vi "optionsAcq_gainOpticalDetector.vi"(0 "reference":refnum<class "OSA300.lvclass">, 2 "gain_idx":u16=1, 4 "readWrite":enum16{"read", "write"}(ring), 5 "error in (no error)":errorcluster, 7 "ignore range violation (false)":bool) -> (14 "duplicate reference":refnum<class "OSA300.lvclass">, 15 "status":string, 16 "gain_idx  out":u16, 17 "gain_relative":dbl, 19 "error out":errorcluster)   [LabVIEW 2010, in "OSA300.lvclass"]
uses:
  OSA300.lvclass
  _OSAchannel_class/OSAchannel.lvclass
  OSA.lvclass
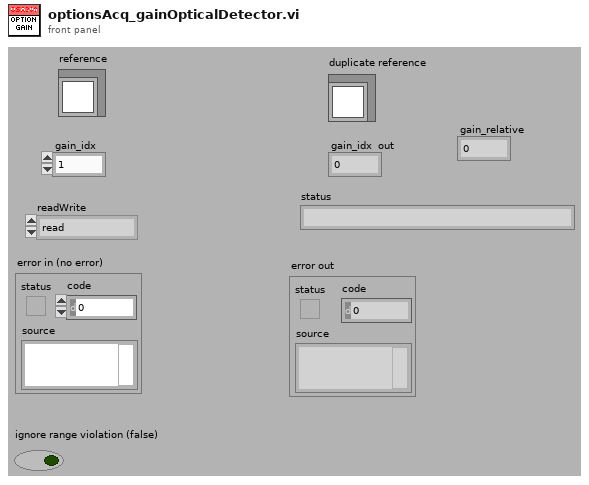
[diagram p1: front panel]
types:
  T1 = typedef "OSA20X_misc.lvlib/amplifier_sort.ctl" = enum16{"amp_unknown", "amp_se_8", "amp_se_12_lg", "amp_se_12", "amp_se_16", "amp_diff_8", "amp_diff_12_lg", "amp_diff_12_ir", "amp_diff_16", "amp_other", "amp_other_2"}
  T2 = typedef "OSA20X_misc.lvlib/detector_sort.ctl" = enum16{"unknown", "Silicon", "Silicon PIN", "Silicon MPPC", "InGaAs", "InGaAs ext low", "InGaAs ext high", "InAs", "InAsSb", "InSb", "MCT", "other", "other2", "other3"}
  T3 = typedef "OSA20X_misc.lvlib/interferogram_smoothing.ctl" = enum16{"NONE", "BINOMIAL", "SAVITSKY_GOLAY", "FOURIER", "MOVING_AVERAGE", "GAUSSIAN"}
  T4 = typedef "OSA20X_misc.lvlib/PDTemperatureMode.ctl" = enum16{"cool: better sensitivity/noise floor", "warm: extended wl range"}
  T5 = cluster{"waveMin (cm-1)":sgl, "waveMax (cm-1)":sgl, "gainOffset_auto":bool, "gain":i32, "gain levels nr":u16, "offset":i32, "offset max":u16, "damper available":bool, "damper active":bool, "amplifier sort":T1, "detector sort":T2, "channelIdx global":u16, "spectrIdx":u16, "waveMeter on":bool, "ref gainLevels rel.":refnum<data-value>, "intfgrm_smooth_width":u16, "intfgrm_smooth_nrOfPasses":u16, "intfgrm_smooth":T3, "adc #bits":u16, "temp Variable":bool, "spectr_smooth":T3, "spectr_smooth_width":u16, "spectr_smooth_nrOfPasses":u16, "PD sensitivity mode":T4, "damper auto":bool}
  T6 = typedef "OSA.lvclass/ObjectAttributes.ctl" = cluster{"Stop":bool, "dataType":T7, "spectrometerIdx":u16, "buffer size interferogram":i32, "interferogram":cluster{"new":bool, "plot_x_ min":sgl, "plot_x_max":sgl, "plot_y_min":sgl, "plot_y_max":sgl, "Graph Intrfrgrm":T8, "timeStamp":u32, "signal (%)":dbl, "traces":cluster{"idx":u32, "broadBand":bool, "monoChromatic":bool, "peakToPeakSignal":dbl, "peakToPeakPos":dbl}[], "traces idx last":i32}, "spectrum":cluster{"new":bool, "plot_x_min":sgl, "plot_x_max":sgl, "plot_unit_x":T9, "plot_unit_y":T10, "plot_y_min":sgl, "plot_y_max":sgl, "Graph Spectrum":T8, "timeStamp":u32, "X_VAL_OPTIONS":enum16{"MIN_MAX", "ARRAY"}, "traces":cluster{"idx":u32}[], "traces idx last":i32}, "Thorlabs_OSA_64.lvclass:queue_action.ctlqueue ref":refnum<queue>, "action":T11, "plot zoom step":dbl, "buffer semaphore":T12, "acq stopped":bool, "dataType active":T7, "temperature (degr C)":sgl, "pressure (hPa)":sgl, "rel humidity (%)":sgl, "settings":cluster{"resolution":u16, "sensitivity":u16, "Average":bool, "average nr":u32, "apodisation":T13, "acq delay (ms)":u32, "airMesure":T14, "wmtr on":bool, "intfgrm_smooth_width":u16, "intfgrm_smooth_nrOfPasses":u16, "intfgrm_smooth":T3, "phaseCorrection":T15, "zeroFill":u8, "spectr_smooth":T3, "spectr_smooth_width":u16, "spectr_smooth_nrOfPasses":u16, "resolution (/cm)":sgl, "REF wavelength, (nm)":dbl, "gain_idx":u16, "gainAuto":bool, "gain_relative":dbl, "PD sensitivity mode":T4, "PD senseMode implemented":bool, "SensorTemperature implemented":bool, "SensorPressure implemented":bool, "SensorHumidity implemented":bool, "attenuationAuto":bool, "attenuationOnOff":bool, "attenuationAvailable":bool, "offsetAvailable":bool, "offset":i32, "offset max":u16}, "peaks position":sgl[], "peaks width":sgl[], "peaks height":sgl[], "peaks max nr":u32, "peaks latest nr":i32, "peaks new":bool, "power":dbl, "power new":bool, "path":string, "wavelength (WNr)":dbl, "wavelength new":bool, "buffer size spectrum":i32, "status":string, "vi reference":refnum<vi>, "funcPointer":u64, "libraryPointer":u64, "singleAcquisition":bool, "coherenceLength (cm)":dbl, "coherenceLength new":bool, "spectrometer model":string, "spectrometer serial nr":string, "peaks thld left":sgl[], "peaks thld right":sgl[], "coherenceLength error (cm)":dbl, "ADC bits":u16, "peaks position centroid":sgl[], "peaks height centroid":sgl[], "OSA series":T16, "channel index spectrum":u16, "spectrometer rangeLow, (/cm)":dbl, "spectrometer rangeHigh, (/cm)":dbl, "channel index interferogram":u16}
  T7 = typedef "OSA.lvclass/acq_dataType.ctl" = enum16{"none", "interferogram", "spectrum"}
  T8 = typedef "OSA.lvclass/graph_intensity.ctl" = refnum<vi>
  T9 = typedef "OSA.lvclass/spectrum_x_unit.ctl" = enum16{"wavenr/cm", "THz", "eV", "nm_air", "nm_vac"}
  T10 = typedef "OSA.lvclass/y_unit.ctl" = enum16{"ADC counts", "dBm pwr absolute", "dBm pwr density", "mW pwr absolute", "mW pwr density"}
  T11 = typedef "OSA.lvclass/queue_action.ctl" = enum16{"none", "stop", "GUI_plotInterferogram", "GUI_plotSpectrum", "GUI_plotInterferogramRescale", "GUI_plotSpectrumRescale", "GUI_plotInterferogramReset", "GUI_plotSpectrumReset", "GUI_plotInterferogramAutoScaleY", "GUI_plotSpectrumAutoScaleY", "GUI_plotInterferogramZoomOut", "GUI_plotSpectrumZoomOut", "GUI_plotInterferogramPane", "GUI_plotSpectrumPane", "GUI_plotInterferogramZoomMouse", "GUI_plotSpectrumZoomMouse", "GUI_spectrumChannelType", "GUI_channel", "ENVIRONMENT temperature", "ENVIRONMENT pressure", "MODE_resolution set", "MODE_resolution get", "MODE_sensitivity set", "MODE_sensitivity get", "MODE_PDTemperature set", "MODE_PDTemperature get", "REBOOT/RESET firmware", "ACQASYNC_acquireSingleSpectrum", "ACQASYNC_continuous start", "ACQASYNC_continuous stop\n", "ACQASYNC_get last interferogram", "ACQASYNC_get last spectrum", "ACQASYNC_get last waveNr", "ACQOPT_interferogram smoothing set", "ACQOPT_interferogram smoothing get", "ACQOPT_spectrum smoothing set", "ACQOPT_spectrum smoothing get", "ACQOPT_apodisation type set", "ACQOPT_apodisation type get", "ACQOPT_phase correction type set", "ACQOPT_phase correction type get", "ACQOPT_acqIntervall_set", "ACQOPT_acqIntervall_get", "ACQOPT_average spectrum set", "ACQOPT_average spectrum get", "ACQOPT_rolling average set", "ACQOPT_rolling average get", "ACQOPT_zero fill factor set", "ACQOPT_zero fill factor get", "ACQOPT_cycle counting set", "ACQOPT_cycle counting get", "ACQOPT_air measure option set", "ACQOPT_air measure option get", "ACQOPT_gainLevel auto get", "ACQOPT_gainLevel auto set", "ACQOPT_gainLevel get", "ACQOPT_gainLevel set", "ACQOPT_offset set", "ACQOPT_attenuator_auto_set", "ACQOPT_attenuator_set", "ACQOPT_getAll", "INSTRUMENT_PROPERTY_range_WaveNr_min", "INSTRUMENT_PROPERTY_range_WaveNr_max", "INSTRUMENT_PROPERTY_reference_wavelength_cm^-1", "INSTRUMENT_PROPERTY_samplesPerRefPeriod", "INSTRUMENT_PROPERTY_resolution_waveNrPercm", "INSTRUMENT_PROPERTY_availableGainLevels", "INSTRUMENT_PROPERTY_status", "CONVERT", "ANALYSE_POWER", "ANALYSE_PEAKS", "ANALYSE_WAVELENGTH", "ANALYSE_SPECTRUM", "ANALYSE_INTERFEROGRAM", "ANALYSE_COHERENCE_LENGTH", "MATH", "MATH_power", "MATH_peaks", "FILE", "miscellaneous"}
  T12 = typedef "Semaphore RefNum" = refnum<k1>
  T13 = typedef "OSA.lvclass/apodisation.ctl" = enum16{"NONE", "NORTON_BEER_WEAK", "NORTON_BEER_MEDIUM", "NORTON_BEER_STRONG", "TRIANGULAR", "COSINE", "HANN", "HAMMING", "BLACKMANHARRIS3", "BLACKMANHARRIS4", "GAUSSIAN"}
  T14 = typedef "OSA.lvclass/airMeasure.ctl" = enum16{"TEMPERATURE", "PRESSURE"}
  T15 = typedef "OSA.lvclass/phaseCorrection.ctl" = enum16{"NONE", "MERTZ", "FORMAN", "MERTZ_FILE", "FORMAN_FILE", "FUTURE COMP."}
  T16 = typedef "OSA.lvclass/OSA_series.ctl" = enum16{"OSA200", "OSA300", "UNKNOWN"}
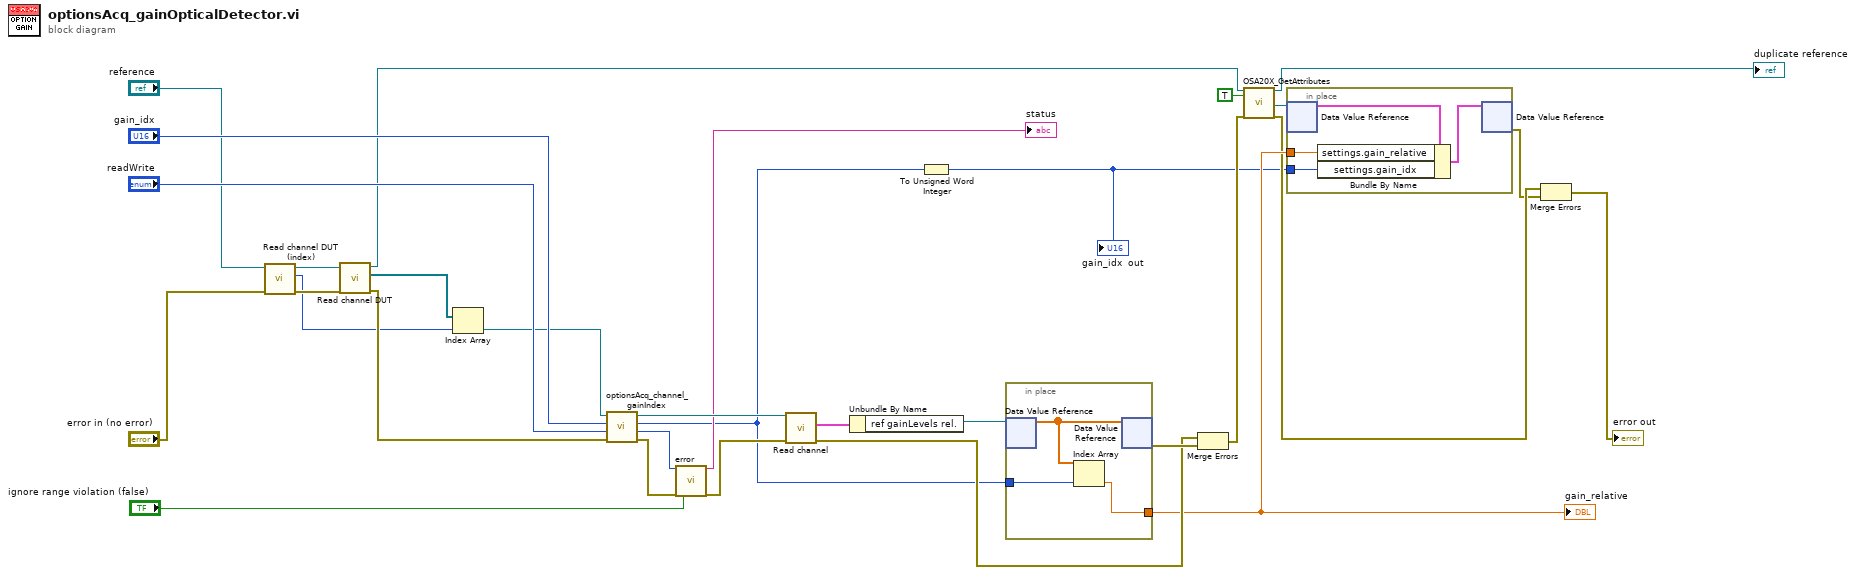
[diagram p0: block diagram]
diagram:
  n1 = call "Read channel DUT (index).vi"("error in (no error)"="error in (no error)", "OSA300 in"="reference") -> ("error out"=w17:errorcluster, "channel ifrgrm (index)"=w12:i32, "OSA300 out"=w14:refnum<class "OSA300.lvclass">)  [unwired: 7 in]
  n2 = call "Read channel DUT.vi"("error in (no error)"=w17, "OSA300 in"=w14) -> ("error out"=w16:errorcluster, "channel DUT"=w13:refnum<class "OSAchannel.lvclass">[], "OSA300 out"=w10:refnum<class "OSA300.lvclass">)  [unwired: 7 in]
  n3 = Index Array(array=w13, index=w12) -> (element=w29:refnum<class "OSAchannel.lvclass">)
  n4 = call "optionsAcq_channel_gainIndex.vi"("error in (no error)"=w16, "readWrite"="readWrite", "gainIndex"="gain_idx", "OSAchannel in"=w29) -> ("error out"=w23:errorcluster, "status_ftsLib"=w21:i32, "gainLevel"=w2:i32, "OSAchannel out"=w28:refnum<class "OSAchannel.lvclass">)  [unwired: 4 in]
  n5 = call "error.vi"("result code"=w21, "error in (no error)"=w23, "ignore range violation"="ignore range violation (false)") -> ("status"=→"status":string, "error out"=w22:errorcluster)  [unwired: 14 in, 1 out]
  n6 = call "Read channel.vi"("error in (no error)"=w22, "OSAchannel in"=w28) -> ("error out"=w24:errorcluster, "channel"=w27:T5)  [unwired: 7 in, 1 out]
  n7 = Unbundle By Name(w27) -> ("ref gainLevels rel."=w26:refnum<data-value>)
  n8 = To Unsigned Word Integer(number=w2) -> (unsigned 16bit integer=w1:u16)
  "gain_idx  out" <- w1
  n9 = in-place {
    in-place-border: w2 -> [w33]
    in-place-border: [w32] -> w8
    n10 = in-place-dvr #1(w26) -> (w34:dbl[])  [unwired: 1 out]
    n11 = Index Array(array=w34, index=w33) -> (element=w32:dbl)
    n12 = in-place-dvr #1(w34) -> (w25:errorcluster)  [unwired: 1 out]
  }
  "gain_relative" <- w8
  n13 = Merge Errors(w24, w25) -> (w7:errorcluster)
  n14 = call "OSA20X_GetAttributes.vi"("reference in"=w10, "OnlyGetDvrReference(False)"=TRUE, "error in (no error)"=w7) -> ("reference out"=→"duplicate reference":refnum<class "OSA300.lvclass">, "DataRef"=w9:refnum<data-value>, "error out"=w5:errorcluster)  [unwired: 13 in, 1 out]
  n15 = in-place {
    in-place-border: w8 -> [w37]
    in-place-border: w1 -> [w35]
    n16 = in-place-dvr #2(w9) -> (w38:T6)  [unwired: 1 out]
    n17 = Bundle By Name(cluster=w38, "settings.gain_relative"=w37, "settings.gain_idx"=w35) -> (w36:T6)
    n18 = in-place-dvr #2(w36) -> (w4:errorcluster)  [unwired: 1 out]
  }
  n19 = Merge Errors(w5, w4) -> (→"error out":errorcluster)
